vi "SCMP - Run Cbk dispaly refesh2.vi"(7 "Function":enum16{"Init", "Update", "Stop"}(ring), 10 "Refresh Time {ms}":u32=1200) -> (2 "Display Refresh":bool)   [LabVIEW 2014]
panel:
  out "Actual time":u32
  out "Next refresh":u32
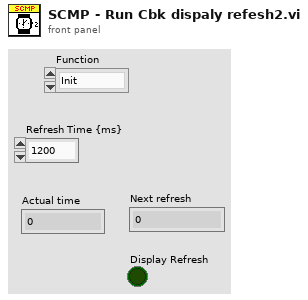
[diagram p1: front panel]
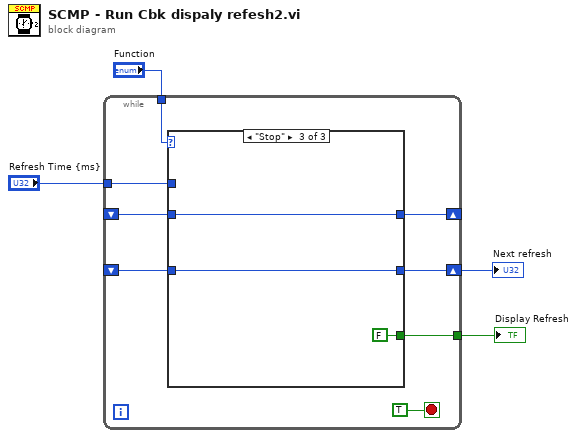
[diagram p0: block diagram]
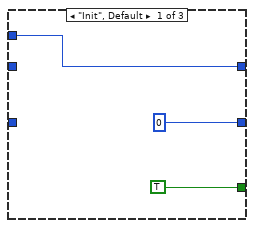
[diagram p2: hidden frame]
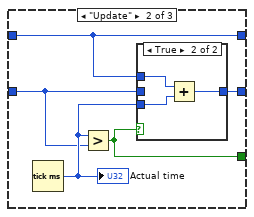
[diagram p3: hidden frame]
diagram:
  n1 = while {
    shift-right: [w12] -> w2
    shift-left: _ -> [w5]
    tunnel: "Refresh Time {ms}" -> [w9]
    tunnel: "Function" -> [w10]
    shift-right: [w8] -> _
    shift-left: _ -> [w7]
    tunnel: [w6] -> w4
    stop <- TRUE stop-if-true
    n2 = case shown="\"Stop\"" w10 {
      tunnel: [TRUE w17 FALSE] -> w6
      tunnel: [u32 0 w20 w26] -> w12
      tunnel: w9 -> [w13 _ _]
      tunnel: [w13 w19 w27] -> w8
      tunnel: w7 -> [_ w19 w27]
      tunnel: w5 -> [_ w16 w26]
      frame "Init", Default {
      }
      frame "Update" {
        n3 = Tick Count (ms)() -> (millisecond timer value=w18:u32)
        "Actual time" <- w18
        n4 = Greater?(x=w18, y=w16) -> (0:w17:bool)
        n5 = case shown="True" w17 {
          tunnel: [w21 w24] -> w20
          tunnel: w19 -> [_ w23]
          tunnel: w18 -> [_ w22]
          tunnel: w16 -> [w21 _]
          frame False {
          }
          frame True {
            n6 = Add(x=w23, y=w22) -> (x+y=w24:u32)
          }
        }
      }
      frame "Stop" {
      }
    }
  }
  "Display Refresh" <- w4
  "Next refresh" <- w2
